vi "tutorial4_boolean.vi"() -> ()   [LabVIEW 2020]
panel:
  out "Boolean":bool
  in  "Tank C":dbl(slide) scale=0.0..10.0
  in  "Tank B":dbl(slide) scale=0.0..10.0
  in  "Tank A":dbl(slide) scale=0.0..10.0
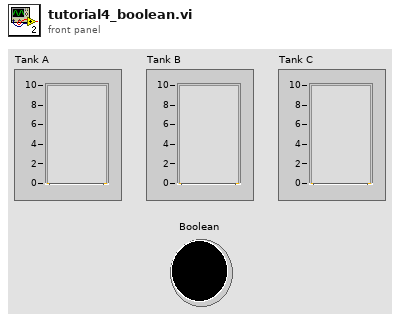
[diagram p1: front panel]
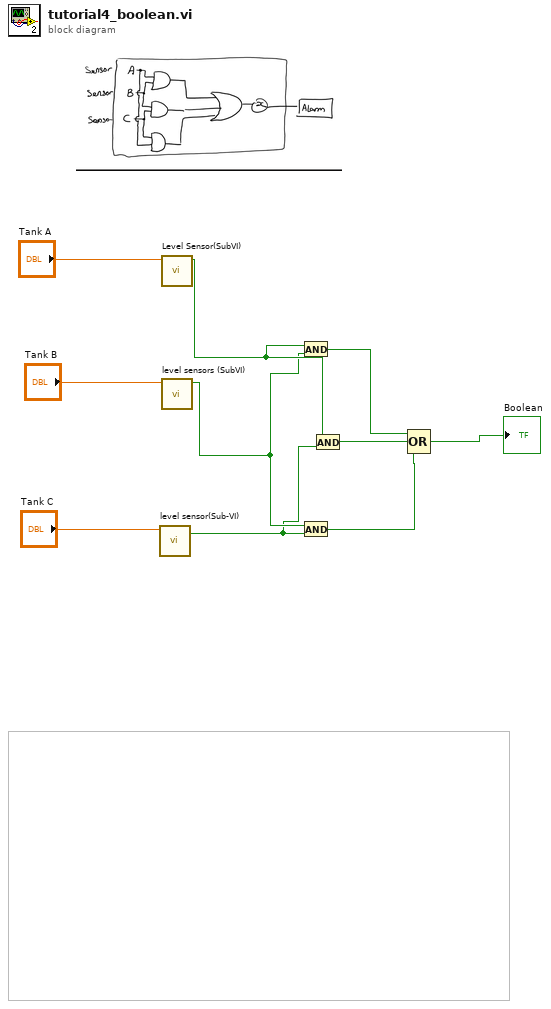
[diagram p0: block diagram]
diagram:
  n1 = call "level sensor(Sub-VI).vi"("Tank C"="Tank C") -> ("Boolean"=w5:bool)  [unwired: 10 in]
  n2 = call "Level Sensor(SubVI).vi"("Tank A"="Tank A") -> ("Boolean"=w7:bool)  [unwired: 10 in]
  n3 = call "level sensors (SubVI).vi"("Tank B"="Tank B") -> ("Boolean"=w6:bool)  [unwired: 10 in]
  n4 = And(x=w7, y=w6) -> (x .and. y?=w4:bool)
  n5 = And(x=w6, y=w5) -> (x .and. y?=w2:bool)
  n6 = And(x=w7, y=w5) -> (x .and. y?=w3:bool)
  n7 = Compound Arithmetic op=OR(w4, w3, w2) -> (→"Boolean":bool)
